vi "DAQ Project VI.vi"() -> ()   [LabVIEW 2016]
uses:
  <vilib>/Analysis/Matrix/Numeric/Conversions/Array To Matrix - RA2.vi
  <vilib>/Analysis/Matrix/NI_Matrix.lvlib
panel:
  in  "Where To Save Data":path
  out "Invalid Entry":bool
  out "Displayed Frequency":dbl
  out "XY Graph":cluster{"Y":dbl[], "Y":dbl[]}[](graph) caption="Gain vs Frequency"
  in  "Upper Frequency (Hz)":dbl=1.0 min=10.0 max=20000.0 step=10.0
  out "Input and Output Voltages":dynamicdata(graph)
  in  "Lower Frequency (Hz)":dbl=10.0 min=10.0 max=20000.0 step=10.0
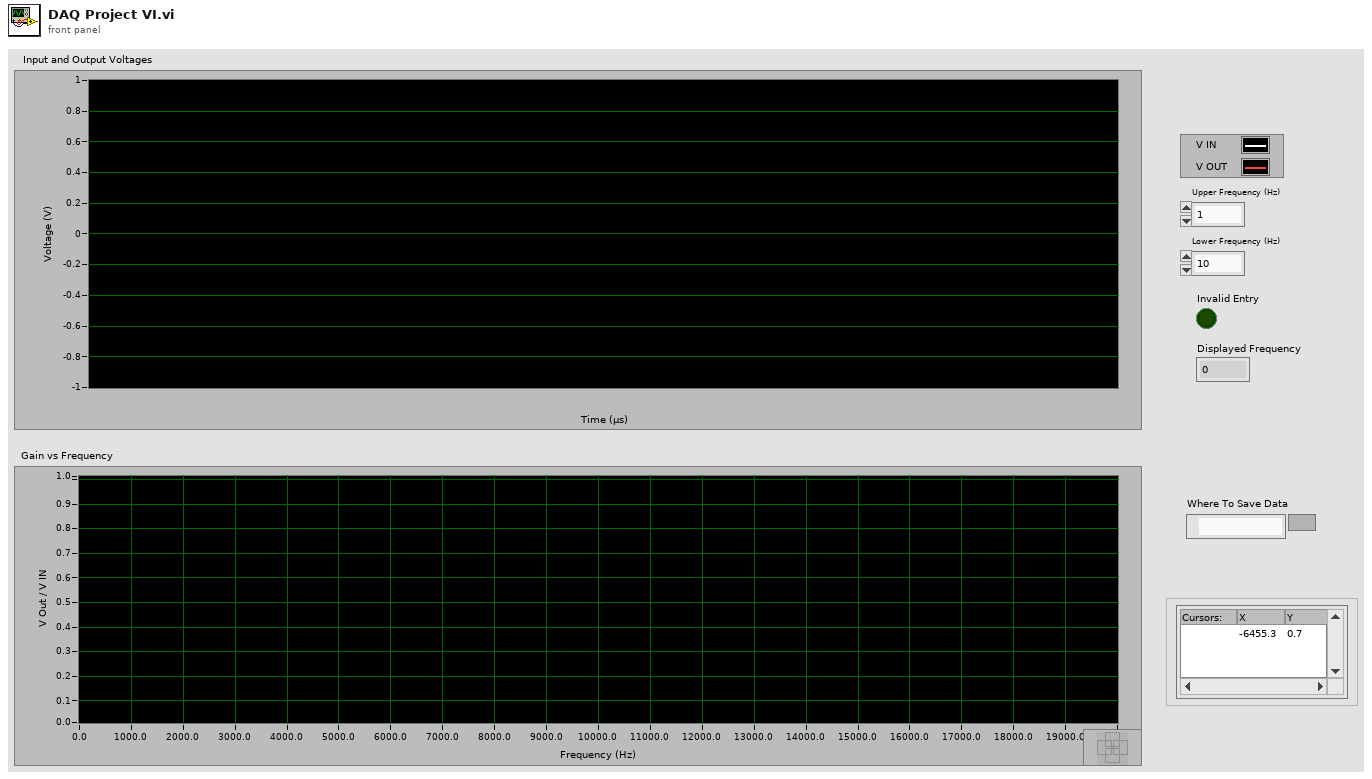
[diagram p1: front panel]
types:
  T1 = typedef "NI_Matrix.lvlib/RealMatrix.ctl" = dbl[][]
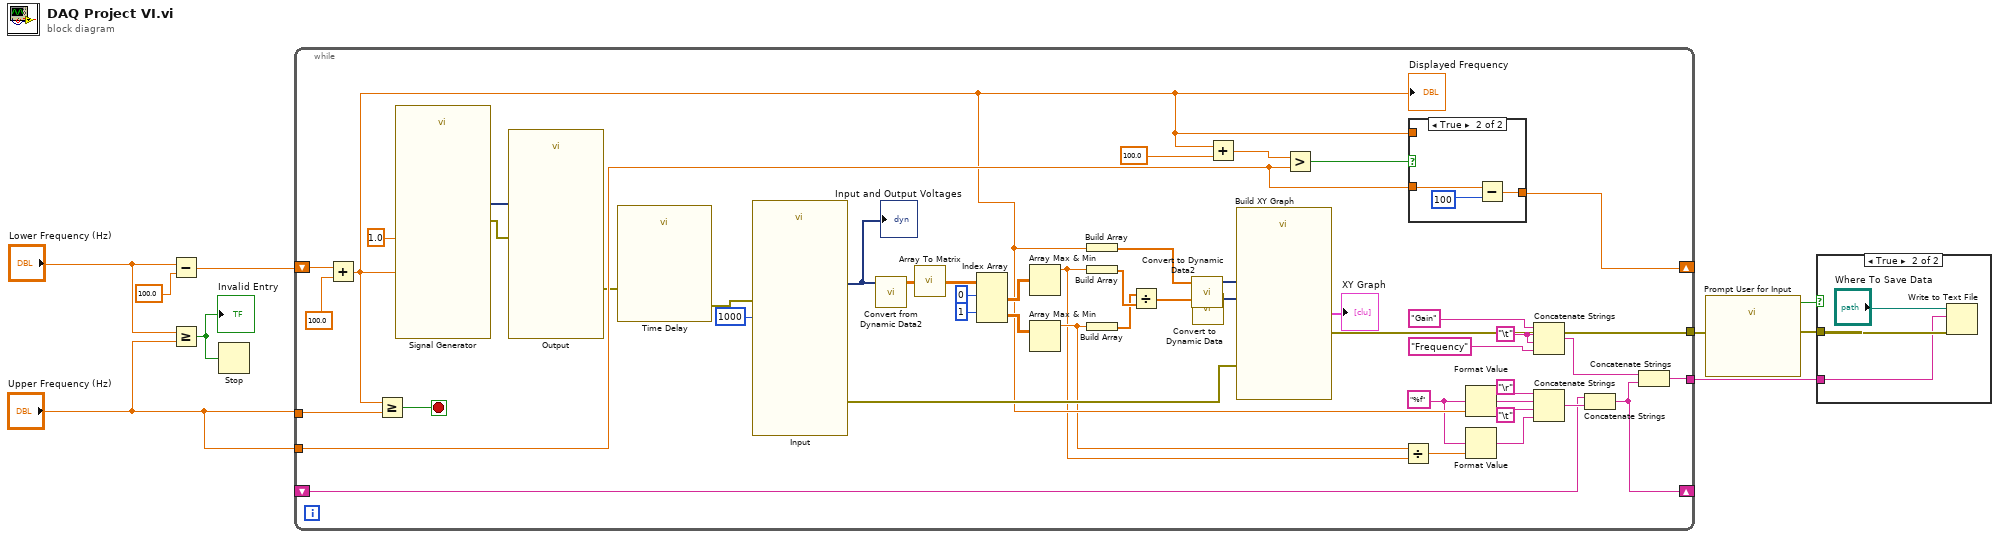
[diagram p0: block diagram]
diagram:
  n1 = Subtract(x="Lower Frequency (Hz)", y=100.0) -> (x-y=w6:dbl)
  n2 = Greater Or Equal?(x="Lower Frequency (Hz)", y="Upper Frequency (Hz)") -> (x >= y?=w8:bool)
  "Invalid Entry" <- w8
  n3 = Stop(stop? (T)=w8) -> ()
  n4 = while {
    shift-right: [w44] -> _
    shift-left: w6 -> [w37]
    tunnel: "Upper Frequency (Hz)" -> [w41]
    tunnel: "Upper Frequency (Hz)" -> [w40]
    shift-right: [w25] -> _
    shift-left: _ -> [w24]
    tunnel: [w17] -> w4
    tunnel: [w10] -> w2
    stop <- w36 stop-if-true
    w14 = "\t"
    w13 = "%f" ("format string")
    n5 = Add(x=w37, y=100.0 ("Frequency Increments")) -> (x+y=w21:dbl)
    "Displayed Frequency" <- w21
    n6 = Greater Or Equal?(x=w21, y=w41) -> (x >= y?=w36:bool)
    n7 = call "Signal Generator"("Frequency"=w21, "Amplitude"=1.0) -> ("Sine"=w57:dynamicdata, "error out"=w56:errorcluster)  [unwired: 12 in]
    n8 = call "Output"("data"=w57, "error in"=w56) -> ("error out"=w39:errorcluster)  [unwired: 15 in, 2 out]
    n9 = call "Time Delay"("error in (no error)"=w39) -> ("error out"=w38:errorcluster)  [unwired: 10 in]
    n10 = call "Input"("number of samples"=1000 ("Number of Samples"), "error in"=w38) -> ("data"=w54:dynamicdata, "error out"=w35:errorcluster)  [unwired: 15 in, 1 out]
    "Input and Output Voltages" <- w54
    n11 = call "Convert from Dynamic Data2"("Dynamic Data Type"=w54) -> ("Array"=w53:dbl[][])  [unwired: 3 in]
    n12 = call-poly <vilib>:"Array To Matrix.vi"("Real 2D Array"=w53) -> ("Real Matrix"=w52:T1)
    n13 = Index Array(array=w52, index (row) #1=0 ("index (row)"), index (row) #2=1 ("index (row)")) -> (element #1=w49:T1, element #2=w48:T1)  [unwired: 2 in]
    n14 = Array Max & Min(array=w49) -> (max value=w19:dbl)  [unwired: 3 out]
    n15 = Array Max & Min(array=w48) -> (max value=w20:dbl)  [unwired: 3 out]
    n16 = Build Array(w21) -> (w22:dbl[])
    n17 = Build Array(w19) -> (w46:dbl[])
    n18 = Build Array(w20) -> (w45:dbl[])
    n19 = Divide(x=w45, y=w46) -> (x/y=w23:dbl[])
    n20 = call "Convert to Dynamic Data2"("Array"=w22) -> ("Dynamic Data Type"=w11:dynamicdata)  [unwired: 3 in]
    n21 = call "Convert to Dynamic Data"("Array"=w23) -> ("Dynamic Data Type"=w12:dynamicdata)  [unwired: 3 in]
    n22 = Add(x=w21, y=100.0) -> (x+y=w43:dbl)
    n23 = call "Build XY Graph"("error in (no error)"=w35, "Y Input"=w12, "X Input"=w11) -> ("error out"=w10:errorcluster, "XY Graph"=→"XY Graph":cluster{"X":dbl[], "Y":dbl[]}[])  [unwired: 7 in]
    n24 = Greater?(x=w43, y=w40) -> (0:w42:bool)
    n25 = Divide(x=w20, y=w19) -> (x/y=w18:dbl)
    n26 = case shown="True" w42 {
      tunnel: w21 -> [w58 _]
      tunnel: [w58 w59] -> w44
      tunnel: w40 -> [_ w61]
      frame False {
      }
      frame True {
        n27 = Subtract(x=w61, y=100) -> (x-y=w59:dbl)
      }
    }
    n28 = Format Value(format string=w13, value (0)=w21) -> (output string=w31:string)  [unwired: 1 in]
    n29 = Format Value(format string=w13, value (0)=w18) -> (output string=w16:string)  [unwired: 1 in]
    n30 = Concatenate Strings("Gain" ("format string"), w14, w14, "Frequency" ("format string")) -> (w27:string)
    n31 = Concatenate Strings("\r", w31, "\t", w16) -> (w30:string)
    n32 = Concatenate Strings(w24, w30) -> (w25:string)
    n33 = Concatenate Strings(w27, w25) -> (w17:string)
  }
  n34 = call "Prompt User for Input"("error in (no error)"=w2) -> ("Save Data File?"=w3:bool, "error out"=w1:errorcluster)  [unwired: 16 in, 1 out]
  n35 = case shown="True" w3 {
    tunnel: w1 -> [_ w64]
    tunnel: w4 -> [_ w62]
    frame False {
    }
    frame True {
      n36 = Write to Text File(file (use dialog)="Where To Save Data", text=w62, error in=w64) -> ()  [unwired: 1 in, 3 out]
    }
  }
